vi "Clicked Report Data.vi"(8 "error in (no error)":errorcluster, 10 "Data":string[][](array[string]), 11 "Table":string) -> (0 "error out":errorcluster)   [LabVIEW 2020]
uses:
  <vilib>/Utility/miscctls.llb/LVRowAndColumnTypeDef.ctl
panel:
  in  "Exit":bool
  in  "Clicked Data":i32(listbox)
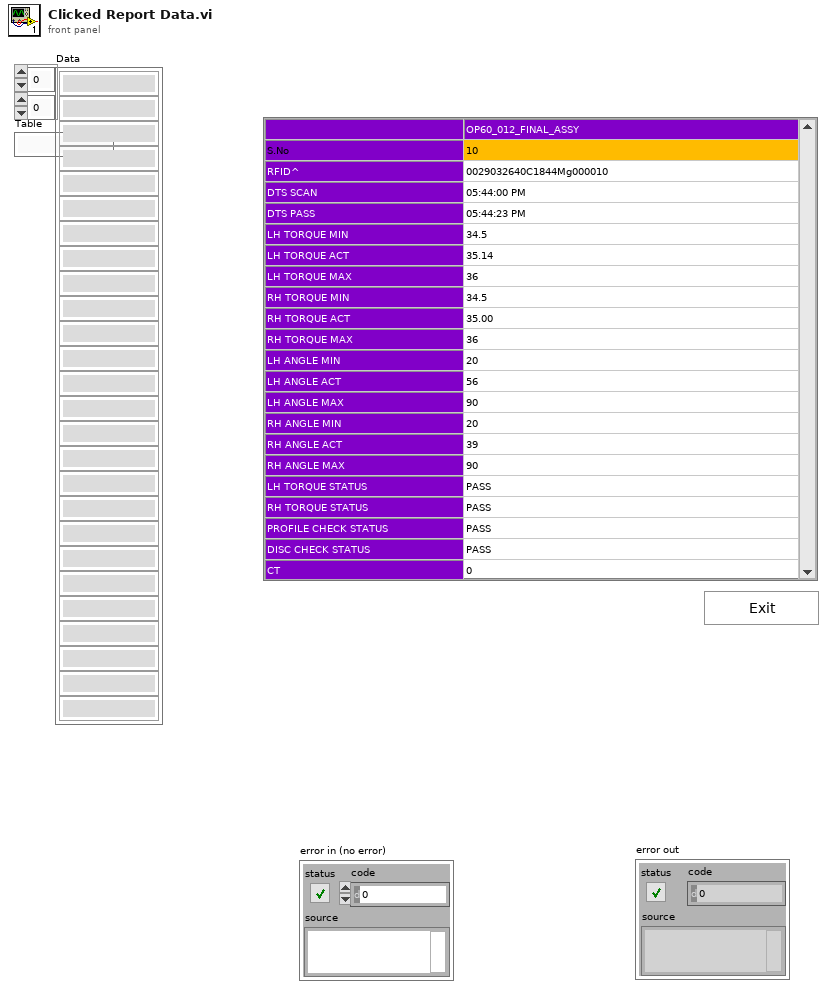
[diagram p1: front panel]
types:
  T1 = typedef "LVRowAndColumnTypeDef.ctl" = cluster{"Row":i32, "Column":i32}
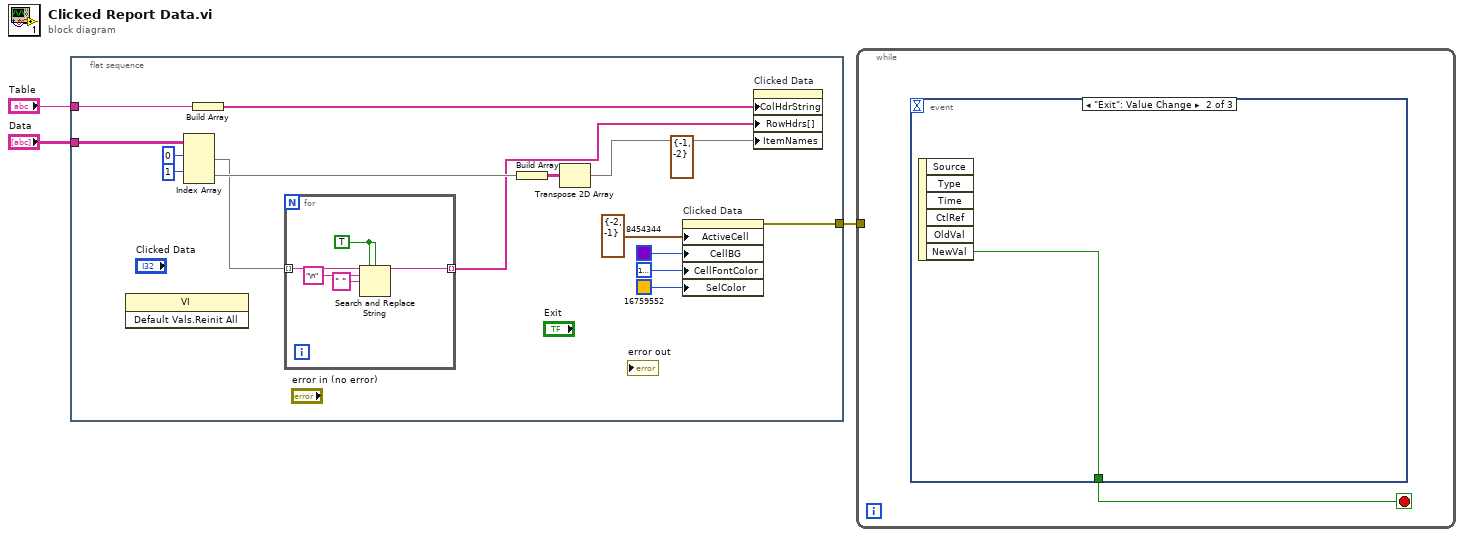
[diagram p0: block diagram]
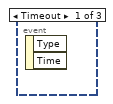
[diagram p2: hidden frame]
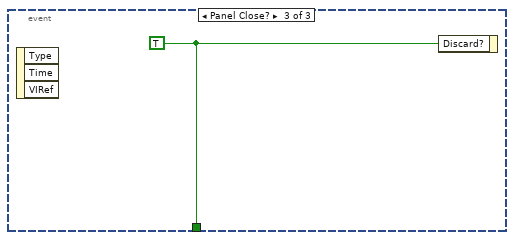
[diagram p3: hidden frame]
diagram:
  n1 = flat-sequence {
    tunnel: [w6] -> w3
    tunnel: "Data" -> [w5]
    tunnel: "Table" -> [w4]
    frame #0 {
      (unwired) T1 {"Row"=-1, "Column"=-2} ("Active Cell:Active Cell")
      n2 = invoke class="VI" method="Default Vals.Reinit All"() -> ()  [unwired: 3 in, 3 out]
      n3 = Index Array(array=w5, index (row) #1=0 ("index (row)"), index (row) #2=1 ("index (row)")) -> (element #1=w8:string[], element #2=w15:string[])  [unwired: 2 in]
      n4 = Build Array(w4) -> (w18:string[])
      n5 = for {
        tunnel: w8 -> [w23] mode=indexing
        tunnel: [w20] -> w7 mode=indexing
        w19 = TRUE ("replace all? (F)")
        n6 = Search and Replace String(replace all?=w19, case sensitive?=w19, input string=w23, search string="\n" ("replace string (\"\")"), replace string=" " ("replace string (\"\")")) -> (result string=w20:string)  [unwired: 3 in, 3 out]
      }
      n7 = Build Array(w15) -> (w14:string[][])
      n8 = Transpose 2D Array(2D array=w14) -> (transposed array=w13:string[][])
      n9 = property on="Clicked Data" class="MCListbox (strict)"("ActiveCell"=T1 {"Row"=-2, "Column"=-1} ("Active Cell:Active Cell"), "CellBG"=u32 8454344 ("Selection Color"), "CellFontColor"=u32 16777226 ("Selection Color"), "SelColor"=u32 16759552 ("Selection Color")) -> (error out=w6:errorcluster)  [unwired: 2 in, 1 out]
      n10 = property on="Clicked Data" class="MCListbox (strict)"("ColHdrString"=w18, "RowHdrs[]"=w7, "ItemNames"=w13) -> ()  [unwired: 2 in, 2 out]
    }
  }
  n11 = while {
    tunnel: w3 -> [_]
    stop <- w24 stop-if-true
    n12 = event shown="[1] \"Exit\": Value Change" {
      selector: _ -> [_ _ _]
      dyn-events: _ -> [_ _ _]
      timeout: _ -> [_ _ _]
      tunnel: [_ w25 w26] -> w24
      event Timeout {
        n13 = event-data() -> ()  [unwired: 1 in, 2 out]
      }
      event "Exit": Value Change {
        n14 = event-data() -> ("NewVal"=w25:bool)  [unwired: 1 in, 5 out]
      }
      event Panel Close? {
        w26 = TRUE ("Discard?")
        n15 = event-data() -> ()  [unwired: 1 in, 3 out]
        n16 = event-data("Discard?"=w26) -> ()  [unwired: 1 in, 1 out]
      }
    }
  }
